vi "global variable-骰寶猜中次數.vi"() -> ()   [LabVIEW 2014]
panel:
  out "»ëÄ_²q¤¤¦¸¼Æ":i32
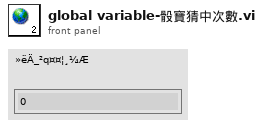
[diagram p1: front panel]
diagram:
